vi "TM response upon error.vi"(9 "error in (no error)":errorcluster, 10 "Command":T1, 11 "Temperature monitor status in in":T2 {"Last update" format="%<%H:%M:%S\n%y/%m/%d>T"}) -> (0 "error out":errorcluster, 1 "Cmd out":T1=enum."Log", 2 "Temperature monitor status out":T2 {"Last update" format="%<%H:%M:%S\n%y/%m/%d>T"}, 3 "Text message":string)   [LabVIEW 2021, in "Temperature monitor.lvlib"]
uses:
  Temperature monitor.lvlib
  Typedefs/TM_status.ctl
  <userlib>/MatS Libs/MatS Mailman/TypeDefs/Mailbox ref.ctl
  Typedefs/TM_commands.ctl
  <userlib>/MatS Libs/MatS Libs.lvlib
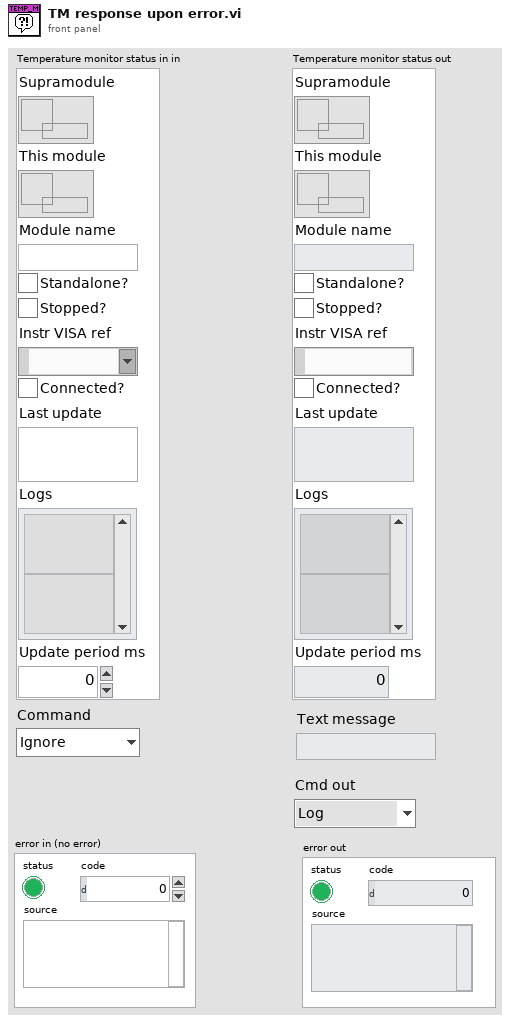
[diagram p1: front panel]
types:
  T1 = typedef "Temperature monitor.lvlib/TM_commands.ctl" = enum16{"Ignore", "Log", "Connect", "Set timeout", "Update", "Disconnect", "End"}
  T2 = typedef "Temperature monitor.lvlib/TM_status.ctl" = cluster{"Supramodule":T3, "This module":T3, "Module name":string, "Standalone?":bool, "Stopped?":bool, "Instr VISA ref":refnum<visa-resource-name>, "Connected?":bool, "Last update":timestamp, "Logs":string[], "Update period ms":u32}
  T3 = typedef "MatS Libs.lvlib/Mailbox ref.ctl" = refnum<queue>
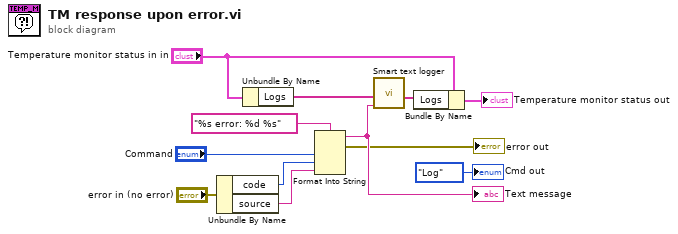
[diagram p0: block diagram]
diagram:
  n1 = Unbundle By Name("error in (no error)") -> ("code"=w6:i32, "source"=w5:string)
  n2 = Unbundle By Name("Temperature monitor status in in") -> ("Logs"=w2:string[])
  n3 = Format Into String(format string="%s error: %d %s" ("f"), "Command", w6, w5) -> (resulting string=w12:string, error out=→"error out":errorcluster)  [unwired: 2 in]
  "Text message" <- w12
  n4 = call <userlib>:"Smart text logger.vi"("Message"=w12, "Logs in"=w2) -> ("Logs out"=w11:string[])  [unwired: 9 in]
  n5 = Bundle By Name(cluster="Temperature monitor status in in", "Logs"=w11) -> (→"Temperature monitor status out":T2)
  "Cmd out" <- TM_commands."Log" ("Cmd out")
